vi "Write udp_refnum.vi"(8 "error in (no error)":errorcluster, 10 "udp_refnum":refnum<k16>, 11 "Socket.UDP in":refnum<class "Socket.UDP.lvclass">) -> (0 "error out":errorcluster, 3 "Socket.UDP out":refnum<class "Socket.UDP.lvclass">)   [LabVIEW 2014, in "Socket.lvlib" / "Socket.UDP.lvclass"]
uses:
  Socket.UDP.lvclass
  Socket.UDP.lvclass/Socket.UDP.ctl
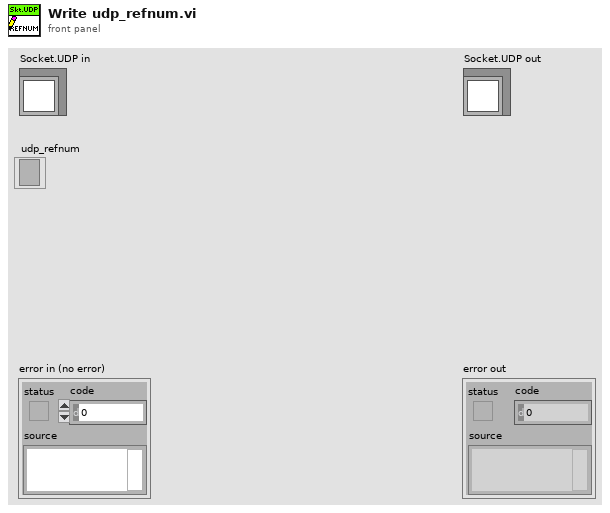
[diagram p1: front panel]
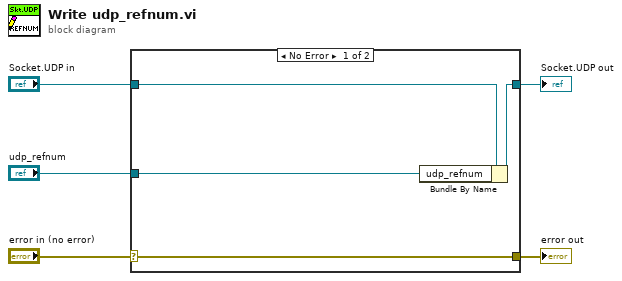
[diagram p0: block diagram]
diagram:
  n1 = case shown="No Error" "error in (no error)" {
    selector: "error in (no error)" -> [w9 w10]
    tunnel: [w9 w10] -> w4
    tunnel: [w7 w11] -> w2
    tunnel: "Socket.UDP in" -> [w8 w11]
    tunnel: "udp_refnum" -> [w6 _]
    frame No Error {
      n2 = Bundle By Name(cluster=w8, "udp_refnum"=w6) -> (w7:refnum<class "Socket.UDP.lvclass">)
    }
    frame Error {
    }
  }
  "error out" <- w4
  "Socket.UDP out" <- w2
